vi "InitDIO.vi"(6 "CardID":u32, 7 "CardName":string, 8 "error in (no error)":errorcluster, 11 "DIO in":refnum<class "DIO.lvclass">) -> (0 "error out":errorcluster, 3 "DIO out":refnum<class "DIO.lvclass">)   [LabVIEW 2024, in "DIO Actor.lvlib" / "DIO.lvclass"]
uses:
  DIO.lvclass
  DIO.lvclass/DIO.ctl
  <userlib>/DAQNavi Polymorphic VI/create/DAQNavi Create Channel(DO-Digital Output).vi
  <userlib>/DAQNavi Polymorphic VI/create/DAQNavi Create Channel(DI-Digital Input).vi
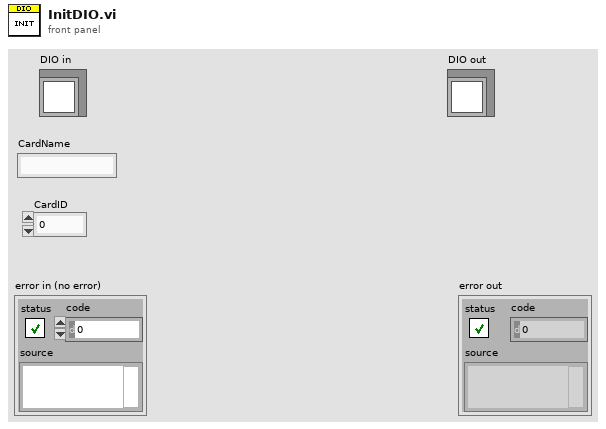
[diagram p1: front panel]
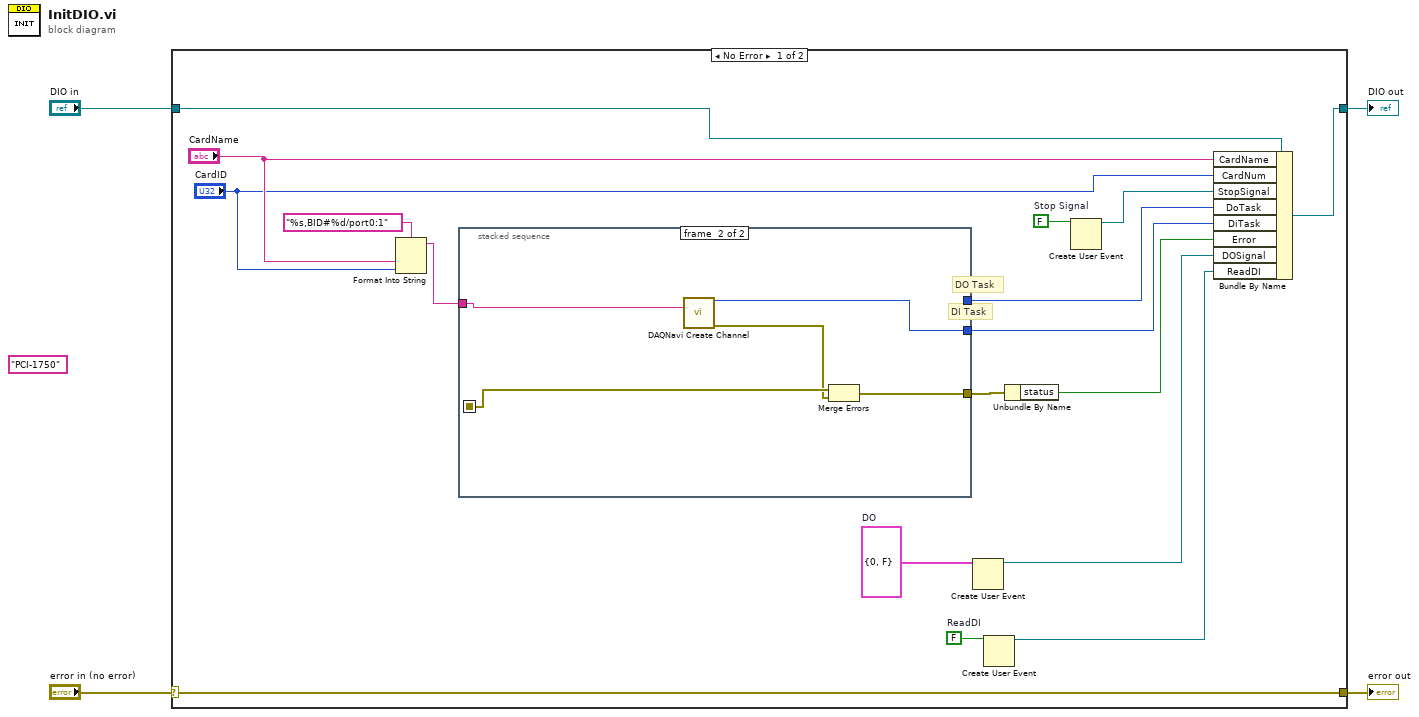
[diagram p0: block diagram]
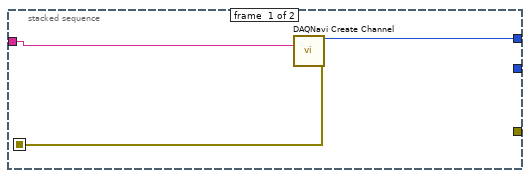
[diagram p2: hidden frame]
diagram:
  (unwired) "PCI-1750" ("regular expression")
  n1 = case shown="No Error" "error in (no error)" {
    selector: "error in (no error)" -> [w19 w31]
    tunnel: [w19 w31] -> w3
    tunnel: [w20 w30] -> w1
    tunnel: "DIO in" -> [w21 w30]
    frame No Error {
      w6 = FALSE  # ReadDI
      w12 = cluster{"Bit":u8, "Value":bool} {"Bit"=0, "Value"=FALSE}  # DO
      w18 = FALSE  # Stop Signal
      # "DI Task"
      # "DO Task"
      n2 = Format Into String(format string="%s,BID#%d/port0:1" ("physical channels"), "CardName", "CardID") -> (resulting string=w7:string)  [unwired: 2 in, 1 out]
      n3 = stacked-sequence {
        seq-local: [w22 _] -> [_ w27]
        tunnel: w7 -> [w24 w29]
        tunnel: [w23 _] -> w15
        tunnel: [_ w28] -> w14
        tunnel: [_ w25] -> w16
        frame #0 {
          n4 = call-poly <userlib>:"DAQNavi Create Channel.vi"("physical channels"=w24) -> ("task out"=w23:i32, "error out"=w22:errorcluster)  [unwired: 13 in]
        }
        frame #1 {
          n5 = call-poly <userlib>:"DAQNavi Create Channel.vi"("physical channels"=w29) -> ("task out"=w28:i32, "error out"=w26:errorcluster)  [unwired: 13 in]
          n6 = Merge Errors(w27, w26) -> (w25:errorcluster)
        }
      }
      n7 = Create User Event(user event datatype=w12) -> (user event=w11:refnum<user-event>)  [unwired: 1 in, 1 out]
      n8 = Create User Event(user event datatype=w6) -> (user event=w5:refnum<user-event>)  [unwired: 1 in, 1 out]
      n9 = Unbundle By Name(w16) -> ("status"=w13:bool)
      n10 = Create User Event(user event datatype=w18) -> (user event=w17:refnum<user-event>)  [unwired: 1 in, 1 out]
      n11 = Bundle By Name(cluster=w21, "CardName"="CardName", "CardNum"="CardID", "StopSignal"=w17, "DoTask"=w15, "DiTask"=w14, "Error"=w13, "DOSignal"=w11, "ReadDI"=w5) -> (w20:refnum<class "DIO.lvclass">)
    }
    frame Error {
    }
  }
  "error out" <- w3
  "DIO out" <- w1
